vi "Fit Data.vi"(8 "error in":errorcluster, 10 "Data In":dbl[](array[numeric]), 11 "Fit Exponential in":refnum<class "Fit Exponential.lvclass">) -> (0 "error out":errorcluster, 3 "Fit Exponential out":refnum<class "Fit Exponential.lvclass">)   [LabVIEW 2014, in "Exponential Fit Library.lvlib" / "Fit Exponential.lvclass"]
uses:
  Fit Exponential.lvclass
  Fit Exponential.lvclass/Fit Exponential.ctl
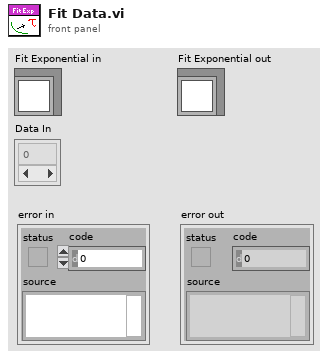
[diagram p1: front panel]
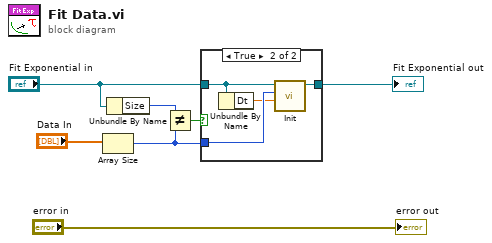
[diagram p0: block diagram]
diagram:
  n1 = Array Size(array="Data In") -> (size(s)=w2:i32)
  n2 = Unbundle By Name("Fit Exponential in") -> ("Size"=w5:i32)
  n3 = Not Equal?(x=w5, y=w2) -> (x != y?=w4:bool)
  n4 = case shown="True" w4 {
    tunnel: "Fit Exponential in" -> [w8 w10]
    tunnel: w2 -> [_ w12]
    tunnel: [w8 w11] -> w1
    frame False {
    }
    frame True {
      n5 = Unbundle By Name(w10) -> ("Dt"=w9:dbl)
      n6 = call-dynamic "Init.vi"("Dt"=w9, "Size"=w12, "Fit Exponential in"=w10) -> ("Fit Exponential out"=w11:refnum<class "Fit Exponential.lvclass">)  [unwired: 8 in]
    }
  }
  "Fit Exponential out" <- w1
  "error out" <- "error in"
